vi "relative access path.vi"(11 "Oauth2.LinkedIn":refnum<class "Oauth2.LinkedIn.lvclass">) -> (1 "Token Access Path":string, 2 "Authorization Path":string)   [LabVIEW 2020, in "Oauth2.LinkedIn.lvclass"]
uses:
  Oauth2.LinkedIn.lvclass
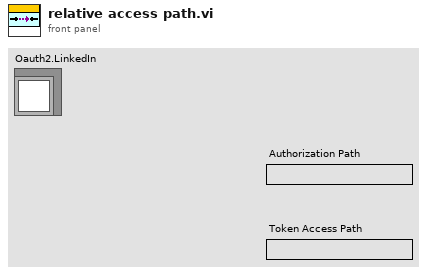
[diagram p1: front panel]
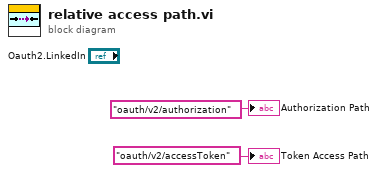
[diagram p0: block diagram]
diagram:
  "Authorization Path" <- "oauth/v2/authorization" ("Authorization Path")
  "Token Access Path" <- "oauth/v2/accessToken" ("Authorization Path")
